vi "AG_Exercise2_Task1.vi"() -> ()   [LabVIEW 2014, in "Gupta_7th.lvrbt"]
uses:
  Gupta_7th.lvrbt
  <vilib>/NXT/Dual Mode Library/Display/drawText.vi
panel:
  out "Result":dbl
  out "A+B":dbl
  in  "B":dbl
  in  "A":dbl
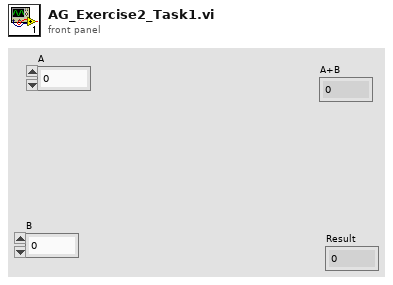
[diagram p1: front panel]
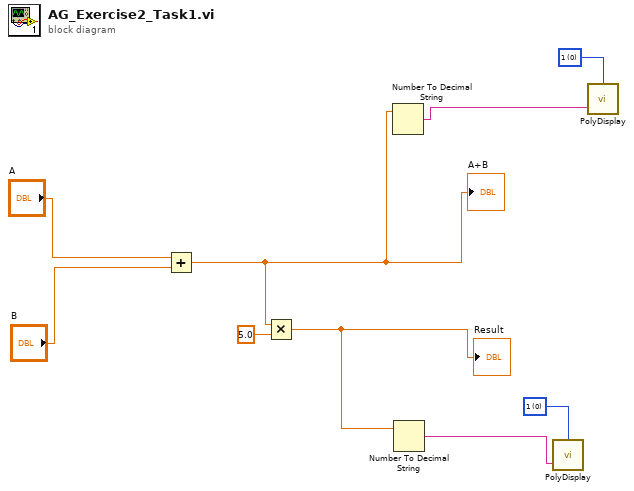
[diagram p0: block diagram]
diagram:
  w2 = i16 0 items=["1", "2", "3", "4", "5", "6", "7", "8", "9", "10", "11", "12"] ("Line")
  w4 = i16 0 items=["1", "2", "3", "4", "5", "6", "7", "8", "9", "10", "11", "12"] ("Line")
  n1 = Add(x="A", y="B") -> (x+y=w6:dbl)
  "A+B" <- w6
  n2 = Multiply(x=w6, y=5.0) -> (x*y=w3:dbl)
  "Result" <- w3
  n3 = Number To Decimal String(number=w6) -> (decimal integer string=w5:string)  [unwired: 1 in]
  n4 = Number To Decimal String(number=w3) -> (decimal integer string=w1:string)  [unwired: 1 in]
  n5 = call-poly <vilib>:"PolyDisplay.vi"("Text"=w1, "Line"=w2) -> ()  [unwired: 2 in, 1 out]
  n6 = call-poly <vilib>:"PolyDisplay.vi"("Text"=w5, "Line"=w4) -> ()  [unwired: 2 in, 1 out]
